vi "Read Ad Buf.vi"(3 "error in (no error)":errorcluster caption="错误输入（无错误）", 4 "num":i32, 5 "databuf":sgl[](array[numeric]), 6 "dev":i32) -> (0 "error out":errorcluster caption="错误输出", 1 "databuf out":sgl[](array[numeric]), 2 "function return":i32)   [LabVIEW 2018, in "恒凯采集卡.lvlib"]
doc: "int Read_AdBuf(int dev,float* databuf,int num);"
uses:
  Usb_Daq_V52_32.dll
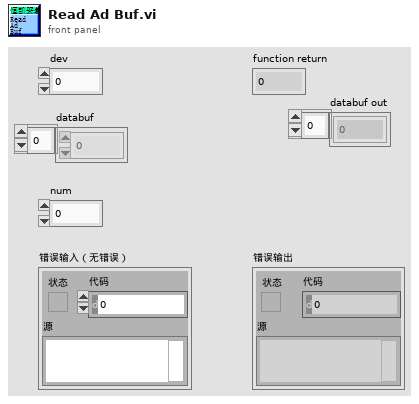
[diagram p1: front panel]
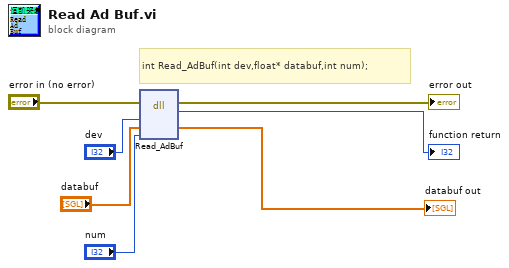
[diagram p0: block diagram]
diagram:
  # "int Read_AdBuf(int dev,float* databuf,int num);"
  n1 = dll-call lib="PTH2Sabs CUsersLenovoDesktop 心肌细胞电信号_231128 -enUsb_Daq_V52_32.*" fn="Read_AdBuf"(error in="error in (no error)", "dev"="dev", "databuf"="databuf", "num"="num") -> (error out=→"error out":errorcluster, "返回类型"=→"function return":i32, "databuf"=→"databuf out":sgl[])  [unwired: 4 in, 1 out]
